vi "Zip.Create Zip Folder with Result and data Files.vi"(8 "error in":errorcluster, 9 "Data Files":path[](array[path]), 10 "Result File":path, 11 "Output Zip File":path) -> (0 "error out":errorcluster)   [LabVIEW 2018]
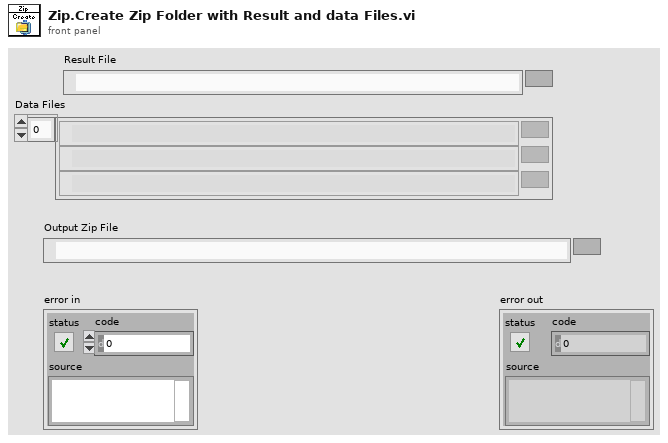
[diagram p1: front panel]
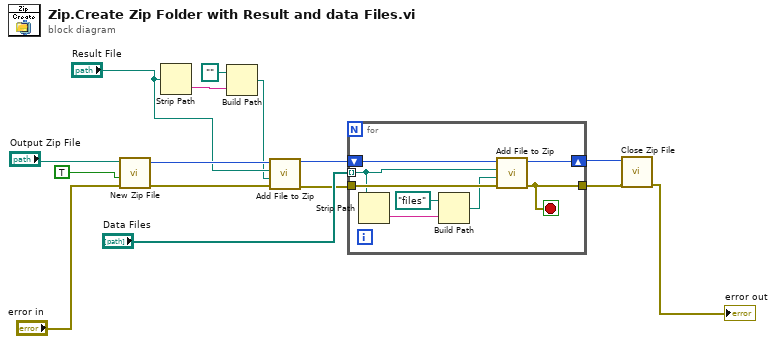
[diagram p0: block diagram]
diagram:
  n1 = call <vilib>:"New Zip File.vi"("error in (no error)"="error in", "confirm overwrite? (F)"=TRUE, "target"="Output Zip File") -> ("error out"=w5:errorcluster, "zip file out"=w6:i64)  [unwired: 2 in, 1 out]
  n2 = Strip Path(path="Result File") -> (name=w8:string)  [unwired: 1 out]
  n3 = Build Path(base path=path "", name or relative path=w8) -> (appended path=w1:path)
  n4 = call <vilib>:"Add File to Zip.vi"("error in (no error)"=w5, "destination path in zip"=w1, "source file path"="Result File", "zip file in"=w6) -> ("error out"=w4:errorcluster, "zip file out"=w3:i64)  [unwired: 6 in]
  n5 = for {
    tunnel: "Data Files" -> [w19] mode=indexing
    tunnel: w4 -> [w22]
    tunnel: [w21] -> w12
    shift-right: [w20] -> w11
    shift-left: w3 -> [w23]
    stop <- w21 stop-if-true
    n6 = Strip Path(path=w19) -> (name=w18:string)  [unwired: 1 out]
    n7 = Build Path(base path=path "files", name or relative path=w18) -> (appended path=w17:path)
    n8 = call <vilib>:"Add File to Zip.vi"("error in (no error)"=w22, "destination path in zip"=w17, "source file path"=w19, "zip file in"=w23) -> ("error out"=w21:errorcluster, "zip file out"=w20:i64)  [unwired: 6 in]
  }
  n9 = call <vilib>:"Close Zip File.vi"("error in (no error)"=w12, "zip file in"=w11) -> ("error out"=→"error out":errorcluster)  [unwired: 5 in]
